vi "Set Display.vi"(8 "error in (no error)":errorcluster, 9 "Channel (T0)":T1 items=["T0", "T1", "A", "B", "C", "D", "E", "F", "G", "H"], 10 "Display Value (Trigger Rate)":i32(ring) items=["Trigger rate", "Trigger threshold", "Trigger single shot", "Trigger line", "Advanced triggering enable", "Trigger holdoff", "Prescale configuration", "Burst mode", "Burst delay", "Burst count", "Burst period", "Channel delay", "Channel output levels", "Channel output polarity", "Burst T0 configuration"], 11 "VISA resource name":refnum<visa-resource-name>) -> (0 "error out":errorcluster, 3 "VISA resource name out":refnum<visa-resource-name>, 4 "Device Errors":cluster{"code":i32, "Text":string}[](array[cluster]))   [LabVIEW 2014, in "Stanford Research DG645 - Driver.lvlib"]
doc: "Status and Display Command: DISP i,c\nInstrument Error Check\n\nSet the display value to i and the displayed channel to c. Parameter c may range from 0-9 for channels T0-H. The parameter i selects the display type.\n\ni Display\n0 Trigger rate\n1 Trigger threshold\n2 Trigger single shot \n3 Trigger line\n4 Advanced triggering enable \n5 Trigger holdoff \n6 Prescale configuration\n7 Burst mode\n8 Burst delay\n8 Burst count\n10 Burst period \n11 Channel delay\n12 Channel output levels\n13 Channel output polarity\n14 Burst T0 configuration"
uses:
  Stanford Research DG645 - Driver.lvlib
  Channel.ctl
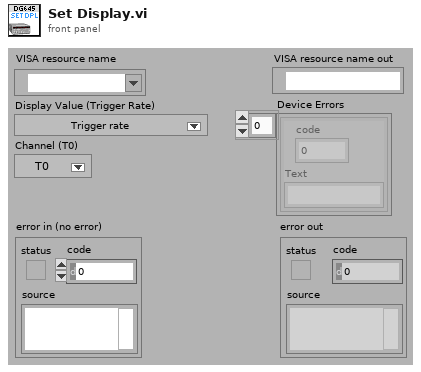
[diagram p1: front panel]
types:
  T1 = typedef "Stanford Research DG645 - Driver.lvlib/Channel.ctl" = i32
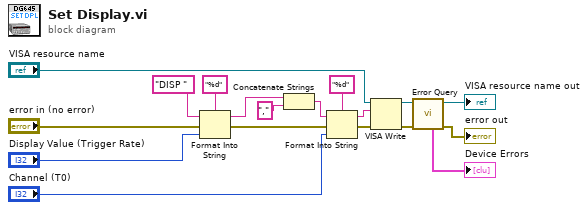
[diagram p0: block diagram]
diagram:
  n1 = Format Into String(format string="%d", initial string="DISP " ("command"), error in="error in (no error)", "Display Value (Trigger Rate)") -> (resulting string=w14:string, error out=w15:errorcluster)
  n2 = Concatenate Strings(w14, "," ("command")) -> (w7:string)
  n3 = Format Into String(format string="%d", initial string=w7, error in=w15, "Channel (T0)") -> (resulting string=w9:string, error out=w10:errorcluster)
  n4 = VISA Write(VISA resource name="VISA resource name", write buffer=w9, error in (no error)=w10) -> (VISA resource name out=w3:refnum<visa-resource-name>, error out=w5:errorcluster)  [unwired: 1 out]
  n5 = call "Error Query.vi"("error in (no error)"=w5, "VISA resource name"=w3) -> ("error out"=→"error out":errorcluster, "VISA resource name out"=→"VISA resource name out":refnum<visa-resource-name>, "Device Errors"=→"Device Errors":cluster{"code":i32, "Text":string}[])  [unwired: 7 in]
